vi "Atoms to GULP File - Copy.vi"(6 "Title":string, 8 "Potential Details":T1(array[cluster])=[{"Atom 1"="Cd core", "Atom 2"="Te core", "Parameters"=[7.261088, 2.51, 23.9020768], "Range Min (A)"=0.0, "Range Max (A)"=4.518}, {"Atom 1"="Cd core", "Atom 2"="Cd core", "Parameters"=[5.327778, 2.51, 34.9560927], "Range Min (A)"=0.0, "Range Max (A)"=4.518}, {"Atom 1"="Te core", "Atom 2"="Te core", "Parameters"=[8.385745, 2.51, 26.4780396], "Range Min (A)"=0.0, "Range Max (A)"=4.518}], 9 "Potential Used":string(combo)="sw2", 10 "Relaxation Type":string(combo)="conv opti", 11 "Structure":T2={"Structure Name"="CdTe", "Lattice vector a"=[6.615785553057252, 0.0, 0.0], "Lattice vector b"=[0.0, 6.615785553057252, 0.0], "Lattice vector c"=[0.0, 0.0, 6.615785553057252], "Atoms Array"=[{"Atom Name"="Cd", "Positions (Direct)"=[[0.0, 0.0, 0.0], [0.0, 0.5, 0.5], [0.5, 0.0, 0.5], [0.5, 0.5, 0.0]], "Positions (Cartesian)"=[[0.0, 0.0, 0.0], [0.0, 3.307892776528626, 3.307892776528626], [3.307892776528626, 0.0, 3.307892776528626], [3.307892776528626, 3.307892776528626, 0.0]]}, {"Atom Name"="Te", "Positions (Direct)"=[[0.25, 0.25, 0.25], [0.75, 0.75, 0.25], [0.75, 0.25, 0.75], [0.25, 0.75, 0.75]], "Positions (Cartesian)"=[[1.653946388264313, 1.653946388264313, 1.653946388264313], [4.96183916479294, 4.96183916479294, 1.653946388264313], [4.96183916479294, 1.653946388264313, 4.96183916479294], [1.653946388264313, 4.96183916479294, 4.96183916479294]]}], "# of atoms"=8}) -> (3 "GULP File":string)   [LabVIEW 2010]
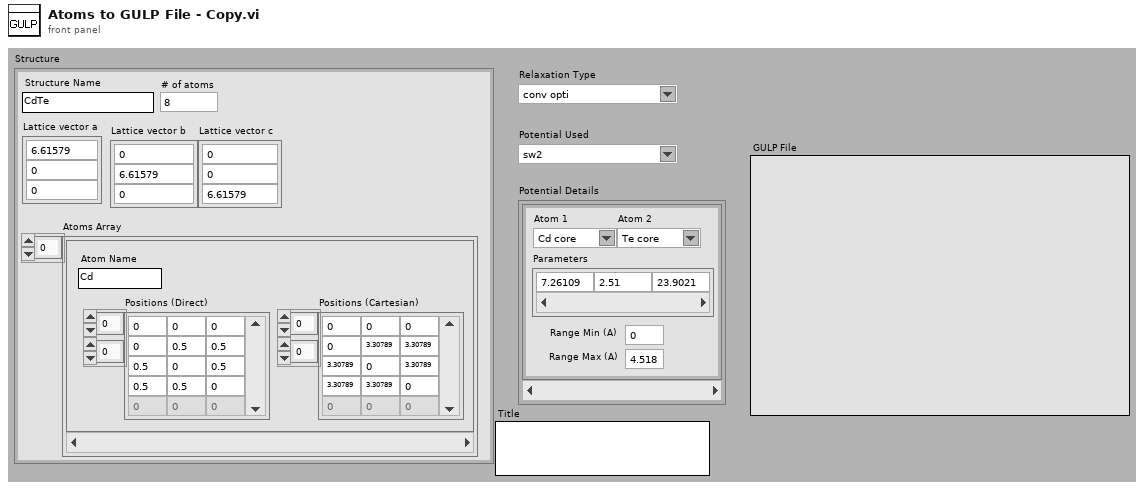
[diagram p1: front panel]
types:
  T1 = cluster{"Atom 1":string, "Atom 2":string, "Parameters":dbl[], "Range Min (A)":dbl, "Range Max (A)":dbl}[]
  T2 = cluster{"Structure Name":string, "Lattice vector a":dbl[], "Lattice vector b":dbl[], "Lattice vector c":dbl[], "Atoms Array":cluster{"Atom Name":string, "Positions (Direct)":dbl[][], "Positions (Cartesian)":dbl[][]}[], "# of atoms":i32}
  T3 = cluster{"Atom Name":string, "Positions (Direct)":dbl[][], "Positions (Cartesian)":dbl[][]}[]
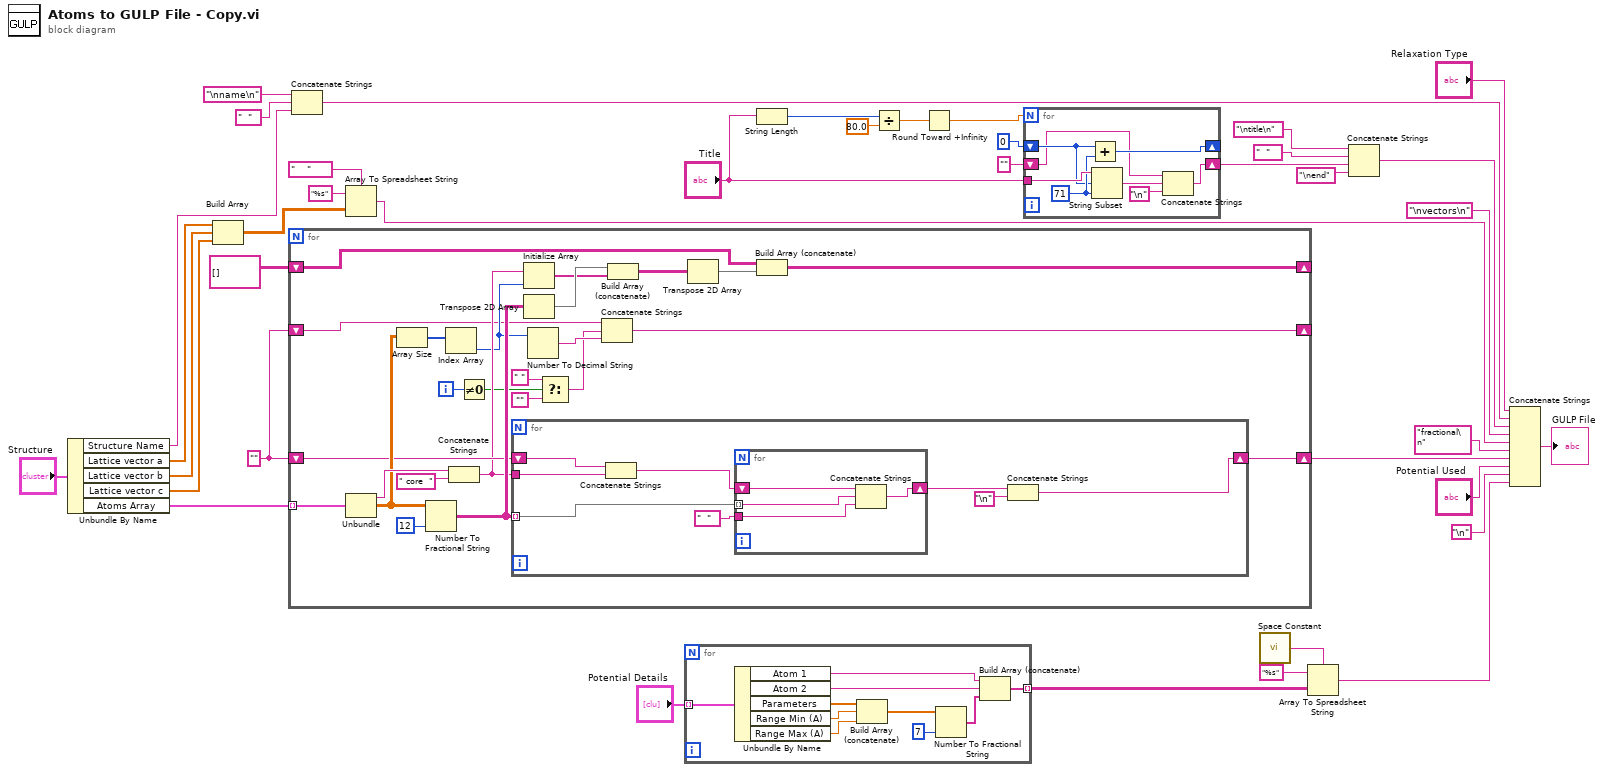
[diagram p0: block diagram]
diagram:
  w38 = ""
  n1 = Unbundle By Name("Structure") -> ("Structure Name"=w15:string, "Lattice vector a"=w35:dbl[], "Lattice vector b"=w34:dbl[], "Lattice vector c"=w33:dbl[], "Atoms Array"=w36:T3)
  n2 = Build Array(w35, w34, w33) -> (w19:dbl[][])
  n3 = for {
    tunnel: w36 -> [w64] mode=indexing
    shift-right: [w61] -> _
    shift-left: string[][] [] -> [w60]
    shift-right: [w53] -> w28
    shift-left: w38 -> [w52]
    shift-right: [w44] -> _
    shift-left: w38 -> [w43]
    i -> [w47]
    n4 = Unbundle(w64) -> ("Atom Name"=w63:string, "Positions (Direct)"=w55:dbl[][])  [unwired: 1 out]
    n5 = Array Size(array=w55) -> (size(s)=w62:i32[])
    n6 = Number To Fractional String(number=w55, precision (6)=i16 12) -> (F-format string=w54:string[][])  [unwired: 2 in]
    n7 = Index Array(array=w62) -> (element=w50:i32)  [unwired: 1 in]
    n8 = Concatenate Strings(w63, " core  " ("string")) -> (w51:string)
    n9 = Not Equal To 0?(x=w47) -> (x != 0?=w49:bool)
    n10 = for {
      tunnel: w54 -> [w72] mode=indexing
      shift-right: [w70] -> w53
      shift-left: w52 -> [w67]
      tunnel: w51 -> [w66]
      n11 = Concatenate Strings(w67, w66) -> (w65:string)
      n12 = for {
        tunnel: w72 -> [w75] mode=indexing
        shift-right: [w74] -> w68
        shift-left: w65 -> [w73]
        tunnel: "  " ("delimiter (Tab)") -> [w76]
        n13 = Concatenate Strings(w73, w75, w76) -> (w74:string)
      }
      n14 = Concatenate Strings(w68, "\n") -> (w70:string)
    }
    n15 = Initialize Array(w51, w50) -> (w58:string[])
    n16 = Transpose 2D Array(2D array=w54) -> (transposed array=w59:string[][])
    n17 = Number To Decimal String(number=w50) -> (decimal integer string=w46:string)  [unwired: 1 in]
    n18 = Select(t=" " ("string"), s=w49, f="") -> (s? t:f=w45:string)
    n19 = Concatenate Strings(w43, w45, w46) -> (w44:string)
    n20 = Build Array (concatenate)(w59, w58) -> (w57:string[][])
    n21 = Transpose 2D Array(2D array=w57) -> (transposed array=w56:string[][])
    n22 = Build Array (concatenate)(w60, w56) -> (w61:string[][])
  }
  n23 = Concatenate Strings("\nname\n" ("string"), "  ", w15) -> (w14:string)
  n24 = Array To Spreadsheet String(delimiter (Tab)="    " ("string"), array=w19, 3:"%s" ("format string")) -> (spreadsheet string=w17:string)
  n25 = for {
    tunnel: "Potential Details" -> [w86] mode=indexing
    tunnel: [w77] -> w24 mode=indexing
    n26 = Unbundle By Name(w86) -> ("Atom 1"=w84:string, "Atom 2"=w83:string, "Parameters"=w81:dbl[], "Range Min (A)"=w80:dbl, "Range Max (A)"=w79:dbl)
    n27 = Build Array (concatenate)(w81, w80, w79) -> (w78:dbl[])
    n28 = Number To Fractional String(number=w78, precision (6)=i16 7) -> (F-format string=w82:string[])  [unwired: 2 in]
    n29 = Build Array (concatenate)(w84, w83, w82) -> (w77:string[])
  }
  n30 = String Length(string="Title") -> (length=w6:i32)
  n31 = Divide(x=w6, y=80.0) -> (x/y=w5:dbl)
  n32 = Round Toward +Infinity(x=w5) -> (ceil(x): smallest int >= x=w4:dbl)
  n33 = for {
    N: w4 -> [_]
    tunnel: "Title" -> [w94]
    shift-right: [w92] -> _
    shift-left: 0 -> [w91]
    shift-right: [w88] -> w1
    shift-left: "" -> [w87]
    w93 = 71 ("length (rest)")
    n34 = Add(x=w91, y=w93) -> (x+y=w92:i32)
    n35 = String Subset(string=w94, offset (0)=w91, length (rest)=w93) -> (substring=w90:string)
    n36 = Concatenate Strings(w87, w90, "\n") -> (w88:string)
  }
  n37 = call <vilib>:"Space Constant.vi"() -> ("String"=w25:string)
  n38 = Array To Spreadsheet String(delimiter (Tab)=w25, array=w24, 3:"%s" ("format string")) -> (spreadsheet string=w23:string)
  n39 = Concatenate Strings("\ntitle\n" ("string"), "  ", w1, "\nend" ("string")) -> (w10:string)
  n40 = Concatenate Strings("Relaxation Type", w14, w10, "\nvectors\n" ("string"), w17, "fractional\n" ("string"), w28, "Potential Used", "\n", w23) -> (→"GULP File":string)
